vi "Write Access.vi"(10 "Access":T1, 11 "Waveform Session in":refnum<class "Waveform Session.lvclass">) -> (3 "Waveform Session out":refnum<class "Waveform Session.lvclass">)   [LabVIEW 2020, in "NI_VS Custom Device Waveform API.lvlib" / "Waveform Session.lvclass"]
uses:
  Waveform Session.lvclass
  Access mode.ctl
  Waveform Session.lvclass/Waveform Session.ctl
  NI_VS Custom Device Waveform API.lvlib
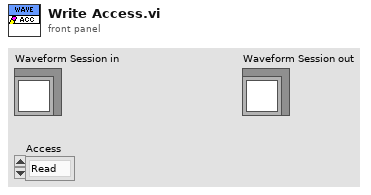
[diagram p1: front panel]
types:
  T1 = typedef "NI_VS Custom Device Waveform API.lvlib/Access mode.ctl" = enum16{"Read", "Write"}
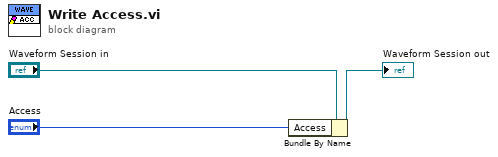
[diagram p0: block diagram]
diagram:
  n1 = Bundle By Name(cluster="Waveform Session in", "Access"="Access") -> (→"Waveform Session out":refnum<class "Waveform Session.lvclass">)
